vi "RandomizeArray_D.vi"(8 "error in (no error)":errorcluster, 11 "Array In":dbl[](array[numeric])) -> (0 "error out":errorcluster, 3 "Array Out":dbl[](array[numeric]))   [LabVIEW 2013]
doc: "Randomizes input array."
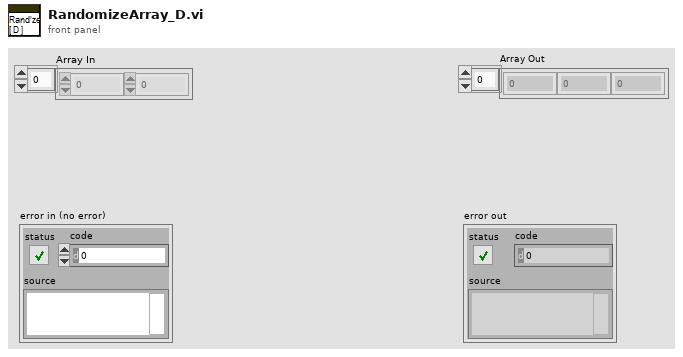
[diagram p1: front panel]
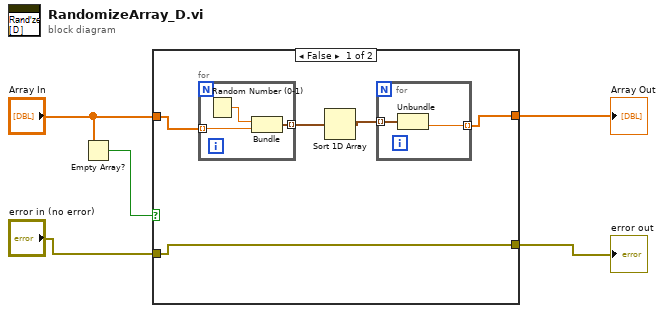
[diagram p0: block diagram]
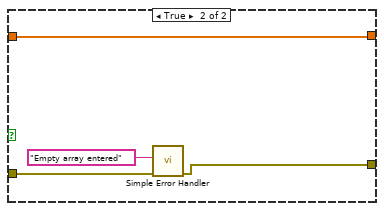
[diagram p2: hidden frame]
diagram:
  n1 = Empty Array?(array="Array In") -> (empty?=w3:bool)
  n2 = case shown="False" w3 {
    tunnel: "error in (no error)" -> [w10 w19]
    tunnel: [w10 w18] -> w4
    tunnel: "Array In" -> [w7 w16]
    tunnel: [w6 w16] -> w1
    frame False {
      n3 = for {
        tunnel: w7 -> [w14] mode=indexing
        tunnel: [w13] -> w9 mode=indexing
        n4 = Random Number (0-1)() -> (number: 0 to 1=w15:dbl)
        n5 = Bundle("number: 0 to 1"=w15, "Numeric"=w14) -> (w13:cluster{"number: 0 to 1":dbl, "Numeric":dbl})  [unwired: 1 in]
      }
      n6 = Sort 1D Array(array=w9) -> (sorted array=w8:cluster{"number: 0 to 1":dbl, "Numeric":dbl}[])
      n7 = for {
        tunnel: w8 -> [w11] mode=indexing
        tunnel: [w12] -> w6 mode=indexing
        n8 = Unbundle(w11) -> ("Numeric"=w12:dbl)  [unwired: 1 out]
      }
    }
    frame True {
      n9 = call <vilib>:"Simple Error Handler.vi"("error source (\" \")"="Empty array entered" ("error source (\" \")"), "error in (no error)"=w19) -> ("error out"=w18:errorcluster)  [unwired: 3 in, 4 out]
    }
  }
  "Array Out" <- w1
  "error out" <- w4
